vi "Start_stopScan.vi"(2 "NMR interval(sec)":dbl, 3 "Count":dbl, 4 "Scan#":i32, 5 "To...(min)":dbl) -> (0 "Stop Scan":dbl format="%#_1g", 1 "StartScan":dbl)   [LabVIEW 2018]
panel:
  out "Start Scan":i32
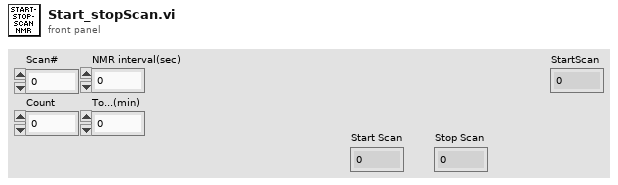
[diagram p1: front panel]
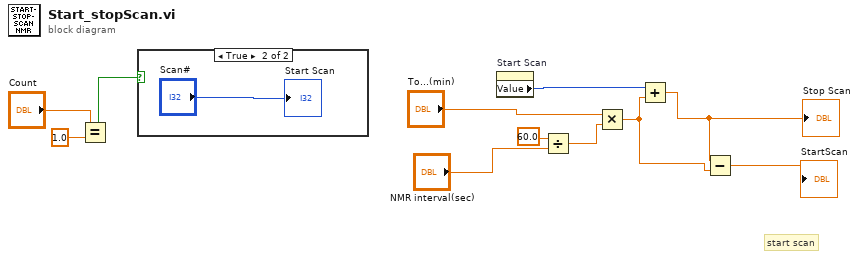
[diagram p0: block diagram]
diagram:
  # "start scan"
  n1 = Equal?(x="Count", y=1.0) -> (x = y?=w11:bool)
  n2 = case shown="True" w11 {
    frame False {
    }
    frame True {
      "Start Scan" <- "Scan#"
    }
  }
  n3 = property on="Start Scan" class="DigNum (strict)"() -> ("Value"=w10:i32)  [unwired: 2 in, 2 out]
  n4 = Divide(x=60.0, y="NMR interval(sec)") -> (x/y=w8:dbl)
  n5 = Multiply(x="To...(min)", y=w8) -> (x*y=w7:dbl)
  n6 = Add(x=w10, y=w7) -> (x+y=w2:dbl)
  "Stop Scan" <- w2
  n7 = Subtract(x=w2, y=w7) -> (x-y=→"StartScan":dbl)
